vi "classes.vi"(0 "HGF_SVFactory":refnum<class "HGF_SVFactory.lvclass">, 1 "className":string, 5 "error in (no error)":errorcluster) -> (14 "dup HGF_SVFactory":refnum<class "HGF_SVFactory.lvclass">, 16 "Object":refnum<class>, 19 "error out":errorcluster)   [LabVIEW 2012, in "HGF_SV.lvlib" / "HGF_SVFactory.lvclass"]
doc: "This dynamaic dispatch VI contains constant objects of all classes that can be produced by HGF_Factory.\n\nChild classes have to override it to define additional classes."
uses:
  HGF_SVFactory.lvclass
  HGF_BaseClasses/HGF_Factory/HGF_Factory.lvclass
  HGF_SVMonitor/HGF_SVMonitor.lvclass
  Visitors/HGF_SVMonitorVisitor/HGF_SVMonitorVisitor.lvclass
  Visitors/HGF_SVMonitorVisitor_register/HGF_SVMonitorVisitor_register.lvclass
  Visitors/HGF_SVMonitorVisitor_deregister/HGF_SVMonitorVisitor_deregister.lvclass
  Visitors/HGF_SVMonitorVisitor_getReg/HGF_SVMonitorVisitor_getReg.lvclass
  Visitors/HGF_SVVarManVisitor_create/HGF_SVVarManVisitor_create.lvclass
  Visitors/HGF_SVVarManVisitor_delete/HGF_SVVarManVisitor_delete.lvclass
  HGF_SVCommand/HGF_SVCommand.lvclass
  HGF_SVSubscriber/HGF_SVSubscriber.lvclass
  HGF_SVService/HGF_SVService.lvclass
  HGF_SVEvent/HGF_SVEvent.lvclass
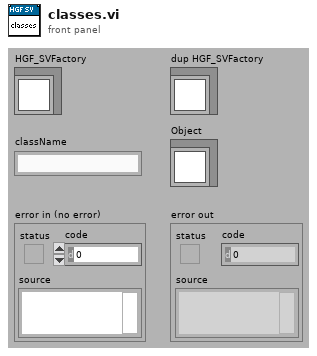
[diagram p1: front panel]
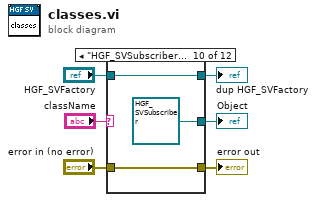
[diagram p0: block diagram]
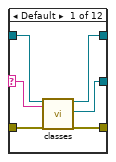
[diagram p2: hidden frame]
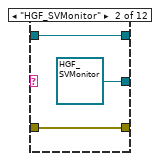
[diagram p3: hidden frame]
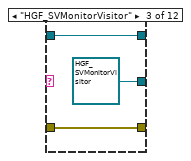
[diagram p4: hidden frame]
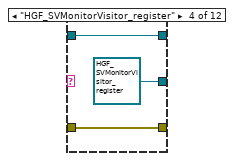
[diagram p5: hidden frame]
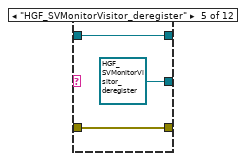
[diagram p6: hidden frame]
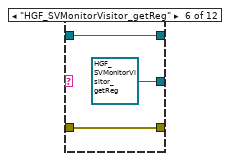
[diagram p7: hidden frame]
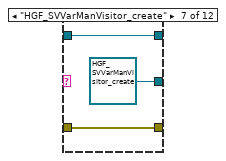
[diagram p8: hidden frame]
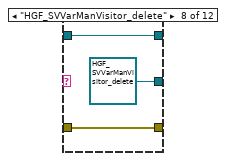
[diagram p9: hidden frame]
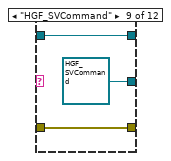
[diagram p10: hidden frame]
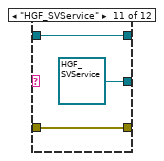
[diagram p11: hidden frame]
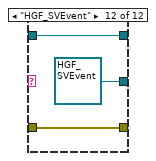
[diagram p12: hidden frame]
diagram:
  n1 = case shown="\"HGF_SVSubscriber\"" "className" {
    selector: "className" -> [w7 _ _ _ _ _ _ _ _ _ _ _]
    tunnel: "HGF_SVFactory" -> [w12 w15 w17 w20 w24 w26 w29 w32 w36 w38 w42 w45]
    tunnel: "error in (no error)" -> [w11 w13 w16 w19 w22 w25 w28 w31 w35 w37 w40 w44]
    tunnel: [w10 w15 w17 w20 w24 w26 w29 w32 w36 w38 w42 w45] -> w4
    tunnel: [w9 refnum<class "HGF_SVMonitor.lvclass"> refnum ("HGF_SV.lvlib:HGF_SVMonitor.lvclass") refnum<class "HGF_SVMonitorVisitor.lvclass"> refnum ("HGF_SV.lvlib:HGF_SVVisitor_runMon.lvclass") refnum<class "HGF_SVMonitorVisitor_register.lvclass"> refnum ("HGF_SV.lvlib:HGF_SVVisitor_register.lvclass") refnum<class "HGF_SVMonitorVisitor_deregister.lvclass"> refnum ("HGF_SV.lvlib:HGF_SVVisitor_deregister.lvclass") refnum<class "HGF_SVMonitorVisitor_getReg.lvclass"> refnum ("HGF_SV.lvlib:HGF_SVMonitorVisitor_getReg.lvclass") refnum<class "HGF_SVVarManVisitor_create.lvclass"> refnum ("HGF_SV.lvlib:HGF_SVVarManVisitor_create.lvclass") refnum<class "HGF_SVVarManVisitor_delete.lvclass"> refnum ("HGF_SV.lvlib:HGF_SVVarManVisitor_delete.lvclass") refnum<class "HGF_SVCommand.lvclass"> refnum ("HGF_SV.lvlib:HGF_SVCommand.lvclass") refnum<class "HGF_SVSubscriber.lvclass"> refnum ("HGF_SV.lvlib:HGF_SVSubscriber.lvclass") refnum<class "HGF_SVService.lvclass"> refnum ("HGF_SV.lvlib:HGF_SVService.lvclass") refnum<class "HGF_SVEvent.lvclass"> refnum ("HGF_SV.lvlib:HGF_SVEvent.lvclass")] -> w3
    tunnel: [w8 w13 w16 w19 w22 w25 w28 w31 w35 w37 w40 w44] -> w2
    frame Default {
      n2 = call-parent "classes.vi"("HGF_Factory"=w12, "className"=w7, "error in (no error)"=w11) -> ("HGF_Factory dup"=w10:refnum<class "HGF_SVFactory.lvclass">, "Object"=w9:refnum<class>, "error out"=w8:errorcluster)  [unwired: 14 out]
    }
    frame "HGF_SVMonitor" {
    }
    frame "HGF_SVMonitorVisitor" {
    }
    frame "HGF_SVMonitorVisitor_register" {
    }
    frame "HGF_SVMonitorVisitor_deregister" {
    }
    frame "HGF_SVMonitorVisitor_getReg" {
    }
    frame "HGF_SVVarManVisitor_create" {
    }
    frame "HGF_SVVarManVisitor_delete" {
    }
    frame "HGF_SVCommand" {
    }
    frame "HGF_SVSubscriber" {
    }
    frame "HGF_SVService" {
    }
    frame "HGF_SVEvent" {
    }
  }
  "error out" <- w2
  "dup HGF_SVFactory" <- w4
  "Object" <- w3
